vi "FunctionGenerator_Add_XY.vi"(9 "X_Y_PAIR":T1 {"Y" format="%_7f"; "X" format="%_7f"}, 11 "in FUNCTION_GENERATOR":T2) -> (3 "out FUNCTION_GENERATOR":T2)   [LabVIEW 2019, in "Trajectory_Library.lvlib"]
doc: "Insert new X, Y pair into an existing Function Generator data cluster.\n\nInputs:\n - \n\nOutputs:\n - Function Generator -- Created data structure"
uses:
  Trajectory_Library.lvlib
  FUNCTION_GENERATOR.ctl
  X_Y_PAIR.ctl
  <vilib>/gmath/interp.llb/Search Ordered Table.vi
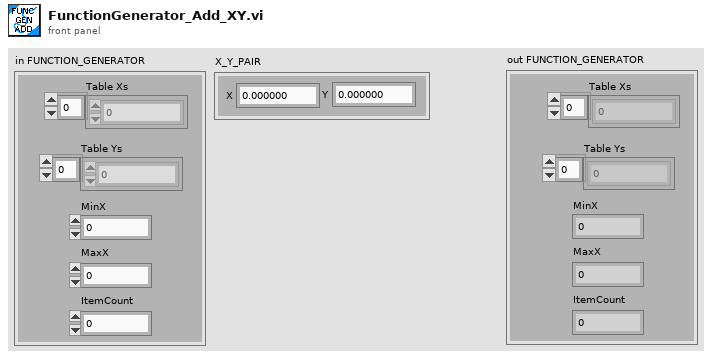
[diagram p1: front panel]
types:
  T1 = typedef "Trajectory_Library.lvlib/X_Y_PAIR.ctl" = cluster{"X":dbl, "Y":dbl}
  T2 = typedef "Trajectory_Library.lvlib/FUNCTION_GENERATOR.ctl" = cluster{"Table Xs":dbl[], "Table Ys":dbl[], "MinX":dbl, "MaxX":dbl, "ItemCount":i32}
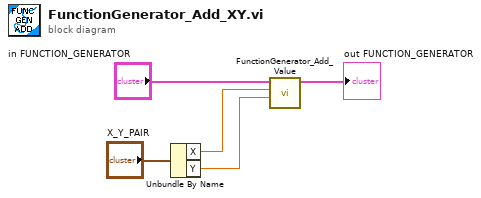
[diagram p0: block diagram]
diagram:
  n1 = Unbundle By Name("X_Y_PAIR") -> ("X"=w2:dbl, "Y"=w1:dbl)
  n2 = call "FunctionGenerator_Add_Value.vi"("Y Value"=w1, "X Value"=w2, "in FUNCTION_GENERATOR"="in FUNCTION_GENERATOR") -> ("out FUNCTION_GENERATOR"=→"out FUNCTION_GENERATOR":T2)  [unwired: 8 in]
